vi "Get Position (SubVI).vi"(8 "error in (no error)":errorcluster, 11 "VISA Refnum in":refnum<visa-resource-name>) -> (0 "error out":errorcluster, 2 "Position":dbl, 3 "VISA Refnum out":refnum<visa-resource-name>)   [LabVIEW 2012]
uses:
  <instrlib>/ZaberTSeries/Public/Utility/Request.ctl
  <instrlib>/ZaberTSeries/ZaberTSeries.lvlib
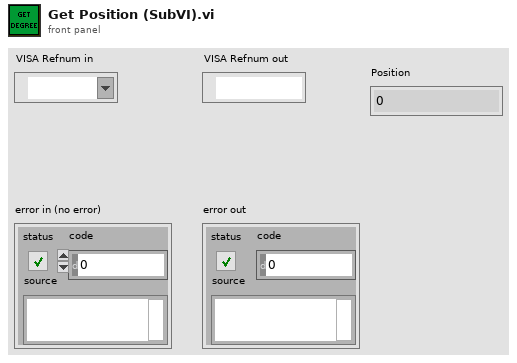
[diagram p1: front panel]
types:
  T1 = typedef "ZaberTSeries.lvlib/Request.ctl" = cluster{"Device Number":u8, "Command":u8, "Data":i32, "Response Count":i32}
  T2 = typedef "ZaberTSeries.lvlib/Response.ctl" = cluster{"Device Number":u8, "Command":u8, "Data":i32}
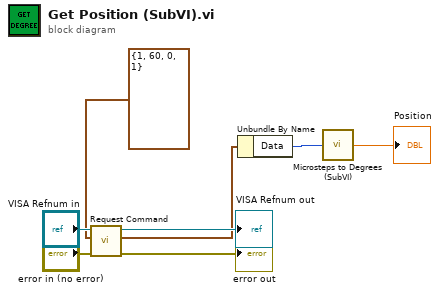
[diagram p0: block diagram]
diagram:
  n1 = call <instrlib>:"Request Command.vi"("error in (no error)"="error in (no error)", "Request"=T1 {"Device Number"=1, "Command"=60, "Data"=0, "Response Count"=1}, "VISA resource name"="VISA Refnum in") -> ("error out"=→"error out":errorcluster, "First Response"=w3:T2, "VISA resource name out"=→"VISA Refnum out":refnum<visa-resource-name>)  [unwired: 5 in, 1 out]
  n2 = Unbundle By Name(w3) -> ("Data"=w2:i32)
  n3 = call "Microsteps to Degrees (SubVI).vi"("Microsteps"=w2) -> ("Numeric"=→"Position":dbl)  [unwired: 4 in]
